vi "Query-Continue-acquisition.vi"(7 "Index":i32, 8 "error in":errorcluster, 9 "Timeout":timestamp, 10 "Acquisition notif":refnum<notifier>, 11 "Acquis. params. ref. in":refnum<data-value>) -> (0 "error IO":errorcluster, 1 "Continue?":bool, 3 "Acquis. params. ref.":refnum<data-value>)   [LabVIEW 2013, in "CameraVision.lvlib" / "CV-Acquisition.lvclass"]
uses:
  CV-Acquisition.lvclass
  CV-Acquisition.lvclass/CV-Acquisition.ctl
  UI/Notifier-with-memory-boolean.vi
  Read Timing source.vi
  Read Acquisition mode.vi
  Read Batch size var.vi
  UI/CV-UI.lvclass
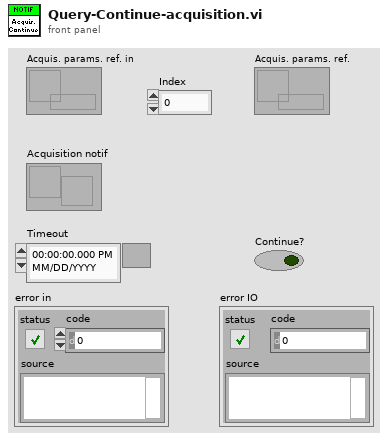
[diagram p1: front panel]
types:
  T1 = enum16{"Continuous", "Continuous batch", "Single batch", "Single batch -delayed"}
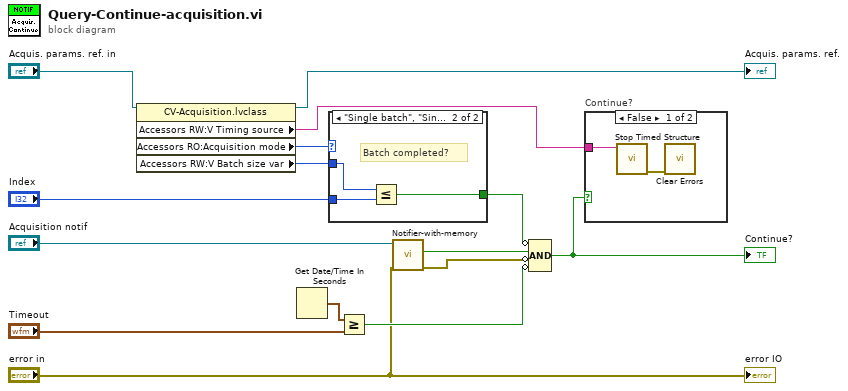
[diagram p0: block diagram]
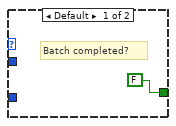
[diagram p3: hidden frame]
diagram:
  n1 = property class="CV-Acquisition.lvclass"(reference="Acquis. params. ref. in") -> (reference out=→"Acquis. params. ref.":refnum<data-value>, "Accessors RW:V Timing source"=w3:string, "Accessors RO:Acquisition mode"=w2:T1, "Accessors RW:V Batch size var"=w1:i32)  [unwired: 1 in, 1 out]
  n2 = Get Date/Time In Seconds() -> (seconds since 1Jan1904=w10:timestamp)
  n3 = case shown="\"Single batch\", \"Single batch -delayed\"" w2 {
    tunnel: w1 -> [_ w19]
    tunnel: "Index" -> [_ w18]
    tunnel: [FALSE w17] -> w9
    frame Default {
      # "Batch completed?"
    }
    frame "Single batch", "Single batch -delayed" {
      # "Batch completed?"
      n4 = Less Or Equal?(x=w19, y=w18) -> (x <= y?=w17:bool)
    }
  }
  n5 = Greater Or Equal?(x=w10, y="Timeout") -> (x >= y?=w6:bool)
  n6 = call-poly "Notifier-with-memory.vi"("error in"="error in", "Notifier in"="Acquisition notif") -> ("error IO"=w7:errorcluster, "Notification"=w8:bool)  [unwired: 8 in]
  n7 = Compound Arithmetic op=AND(invert w9, w8, invert w7, invert w6) -> (w5:bool)
  "Continue?" <- w5
  n8 = case "Continue?" shown="False" w5 {
    tunnel: w3 -> [w21 _]
    frame False {
      n9 = call <vilib>:"Stop Timed Structure.vi"("name"=w21) -> ("error out"=w20:errorcluster)  [unwired: 10 in]
      n10 = call <vilib>:"Clear Errors.vi"("error in (no error)"=w20) -> ()  [unwired: 6 in, 1 out]
    }
    frame True {
    }
  }
  "error IO" <- "error in"
